vi "update_dict_HIS_open.vi"(8 "error in (no error)":errorcluster, 10 "type":string, 11 "dict of HIS IN":variant) -> (0 "error out":errorcluster, 3 "dict of HIS OUT":variant)   [LabVIEW 2015]
uses:
  cluster_template.ctl
  Classes/DATA/HIS/HIS.lvclass
  Classes/DATA/DATA.lvclass/DATA.ctl
  Classes/DATA/DATA.lvclass
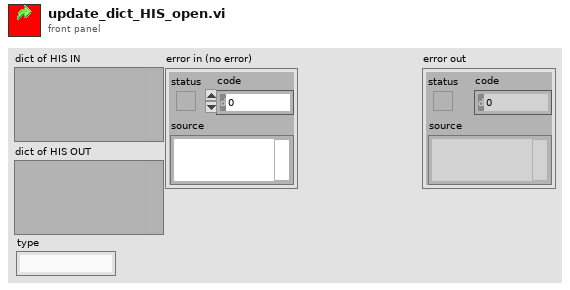
[diagram p1: front panel]
types:
  T1 = typedef "cluster_template.ctl" = cluster{"HIS.lvclass":refnum<class "HIS.lvclass">, "selector":refnum<vi>, "HIS graph":refnum<vi>, "DAT graph":refnum<vi>, "path":refnum<vi>, "path MAIN":refnum<vi>, "#":refnum<vi>, "unsel Graph":refnum<vi>, "DATgraph":refnum<vi>}
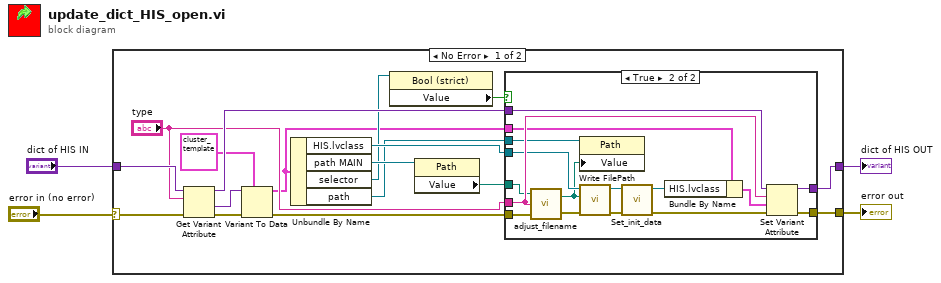
[diagram p0: block diagram]
diagram:
  n1 = case shown="No Error" "error in (no error)" {
    selector: "error in (no error)" -> [w17 w41]
    tunnel: "dict of HIS IN" -> [w21 w40]
    tunnel: [w20 w40] -> w3
    tunnel: [w18 w41] -> w2
    frame No Error {
      n2 = Get Variant Attribute(Variant=w21, name="type", error in=w17) -> (duplicate Variant=w19:variant, value=w16:variant, error out=w15:errorcluster)  [unwired: 1 in, 1 out]
      n3 = Variant To Data(error in=w15, type=T1 {"HIS.lvclass"=refnum, "selector"=refnum, "HIS graph"=refnum, "DAT graph"=refnum, "path"=refnum, "path MAIN"=refnum, "#"=refnum, "unsel Graph"=refnum, "DATgraph"=refnum} ("output cluster"), Variant=w16) -> (data=w6:T1, error out=w14:errorcluster)
      n4 = Unbundle By Name(w6) -> ("HIS.lvclass"=w11:refnum<class "HIS.lvclass">, "path MAIN"=w10:refnum<vi>, "selector"=w8:refnum<vi>, "path"=w5:refnum<vi>)
      n5 = property class="Bool (strict)"(reference=w8) -> ("Value"=w7:bool)  [unwired: 1 in, 2 out]
      n6 = property class="Path"(reference=w10) -> ("Value"=w9:path)  [unwired: 1 in, 2 out]
      n7 = case shown="True" w7 {
        tunnel: [w23 w37] -> w20
        tunnel: w19 -> [w23 w36]
        tunnel: [w22 w35] -> w18
        tunnel: w14 -> [w22 w33]
        tunnel: "type" -> [_ w32]
        tunnel: w11 -> [_ w30]
        tunnel: w9 -> [_ w29]
        tunnel: w6 -> [_ w28]
        tunnel: w5 -> [_ w25]
        frame False {
        }
        frame True {
          n8 = call "adjust_filename.vi"("error in"=w33, "typeIN"=w32, "FilePath IN"=w29) -> ("error out"=w34:errorcluster, "FilePath OUT"=w24:path)
          n9 = property class="Path"(reference=w25, "Value"=w24) -> ()  [unwired: 1 in, 2 out]
          n10 = call "Write FilePath.vi"("error in (no error)"=w34, "FilePath"=w24, "DATA in"=w30) -> ("error out"=w39:errorcluster, "DATA out"=w31:refnum<class "HIS.lvclass">)  [unwired: 7 in]
          n11 = call-dynamic "Set_init_data.vi"("error in (no error)"=w39, "HIS in"=w31) -> ("error out"=w38:errorcluster, "HIS out"=w27:refnum<class "HIS.lvclass">)  [unwired: 8 in]
          n12 = Bundle By Name(cluster=w28, "HIS.lvclass"=w27) -> (w26:T1)
          n13 = Set Variant Attribute(Variant=w36, name=w32, value=w26, error in=w38) -> (Variant out=w37:variant, error out=w35:errorcluster)  [unwired: 1 out]
        }
      }
    }
    frame Error {
    }
  }
  "dict of HIS OUT" <- w3
  "error out" <- w2
